vi "Update Car Wash Entry Indicator.vi"(6 "Vacant?":bool, 11 "Car Wash Display in":refnum<class "Car Wash Display.lvclass">) -> (3 "Car Wash Display out":refnum<class "Car Wash Display.lvclass">)   [LabVIEW 2016, in "CLD Exam - Car Wash.lvlib" / "Car Wash Display.lvclass"]
uses:
  Car Wash Display.lvclass
  Car Wash Display.lvclass/Car Wash Display.ctl
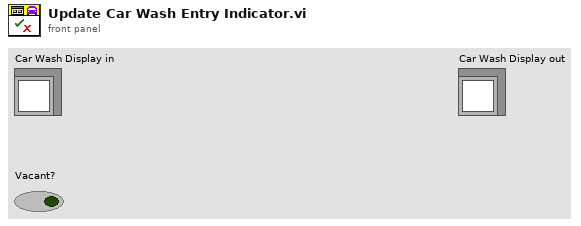
[diagram p1: front panel]
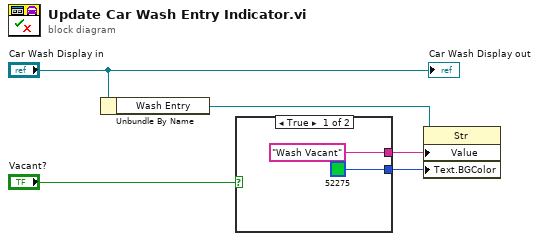
[diagram p0: block diagram]
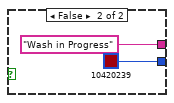
[diagram p2: hidden frame]
diagram:
  n1 = Unbundle By Name("Car Wash Display in") -> ("Wash Entry"=w4:refnum<vi>)
  n2 = case shown="True" "Vacant?" {
    tunnel: [u32 52275 u32 10420239] -> w3
    tunnel: ["Wash Vacant" ("Value") "Wash in Progress" ("Value")] -> w2
    frame True {
    }
    frame False {
    }
  }
  n3 = property class="Str"(reference=w4, "Value"=w2, "Text.BGColor"=w3) -> ()  [unwired: 1 in, 2 out]
  "Car Wash Display out" <- "Car Wash Display in"
